vi "Refresh LabVIEW Menus.vi"(8 "error in (no error)":errorcluster) -> (0 "error out":errorcluster)   [LabVIEW 2017]
doc: "Refreshes the File, Tools, and Help menus."
panel:
  # "Pleasewait while we refresh the LabVIEW File, Tools, and Help menus."
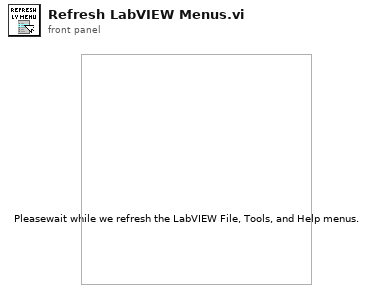
[diagram p1: front panel]
types:
  T1 = enum32{"Invalid", "Standard", "Closed", "Hidden", "Minimized", "Maximized"}
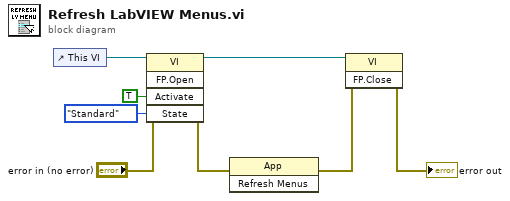
[diagram p0: block diagram]
diagram:
  n1 = control-ref of="This VI"() -> (w8:refnum<vi>)
  n2 = invoke on="Invoke Node" class="VI" method="FP.Open"(reference=w8, error in="error in (no error)", "Activate"=TRUE ("Activate?"), "State"=T1."Standard") -> (reference out=w3:refnum<vi>, error out=w5:errorcluster)  [unwired: 1 in, 3 out]
  n3 = invoke on="Invoke Node" class="App" method="Refresh Menus"(error in=w5) -> (error out=w2:errorcluster)  [unwired: 2 in, 2 out]
  n4 = invoke on="Invoke Node" class="VI" method="FP.Close"(reference=w3, error in=w2) -> (error out=→"error out":errorcluster)  [unwired: 1 in, 2 out]
